vi "Write Index.vi"(8 "error in (no error)":errorcluster, 10 "Index":i32, 11 "DAQmx-Bus_DBLType in":refnum<class "DAQmx-Bus_DBLType.lvclass">) -> (0 "error out":errorcluster, 3 "DAQmx-Bus_DBLType out":refnum<class "DAQmx-Bus_DBLType.lvclass">)   [LabVIEW 2021, in "DAQmx-Bus_DBLType.lvclass"]
uses:
  DAQmx-Bus_DBLType.lvclass
  DAQmx-Bus_DBLType.lvclass/DAQmx-Bus_DBLType.ctl
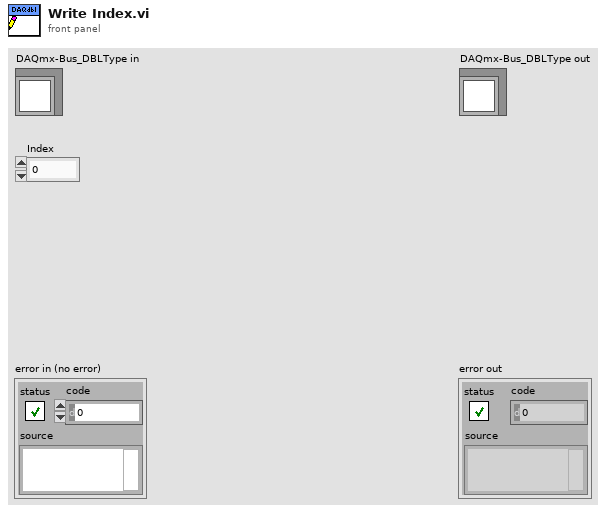
[diagram p1: front panel]
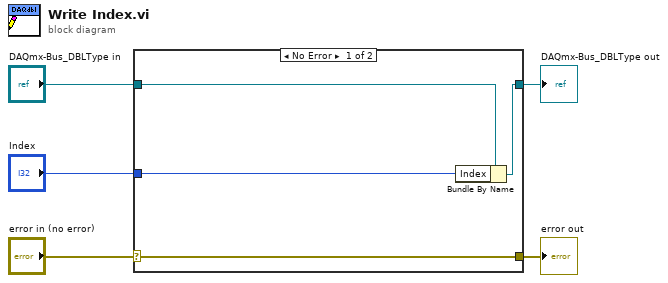
[diagram p0: block diagram]
diagram:
  n1 = case shown="No Error" "error in (no error)" {
    selector: "error in (no error)" -> [w9 w10]
    tunnel: [w9 w10] -> w4
    tunnel: [w7 w11] -> w2
    tunnel: "DAQmx-Bus_DBLType in" -> [w8 w11]
    tunnel: "Index" -> [w6 _]
    frame No Error {
      n2 = Bundle By Name(cluster=w8, "Index"=w6) -> (w7:refnum<class "DAQmx-Bus_DBLType.lvclass">)
    }
    frame Error {
    }
  }
  "error out" <- w4
  "DAQmx-Bus_DBLType out" <- w2
